vi "Edit user.vi"() -> ()   [LabVIEW 2017]
uses:
  <vilib>/Utility/error.llb/DialogType.ctl
  Globle/Cikautxo Intermix Login Details.vi
  Globle/Global 1.vi
panel:
  in  "Remove":bool
  out "error out":errorcluster
  out "Screen Index":i32
  in  "error in (no error)":errorcluster
  in  "User":bool
  in  "Authority":bool
  in  "Home":bool
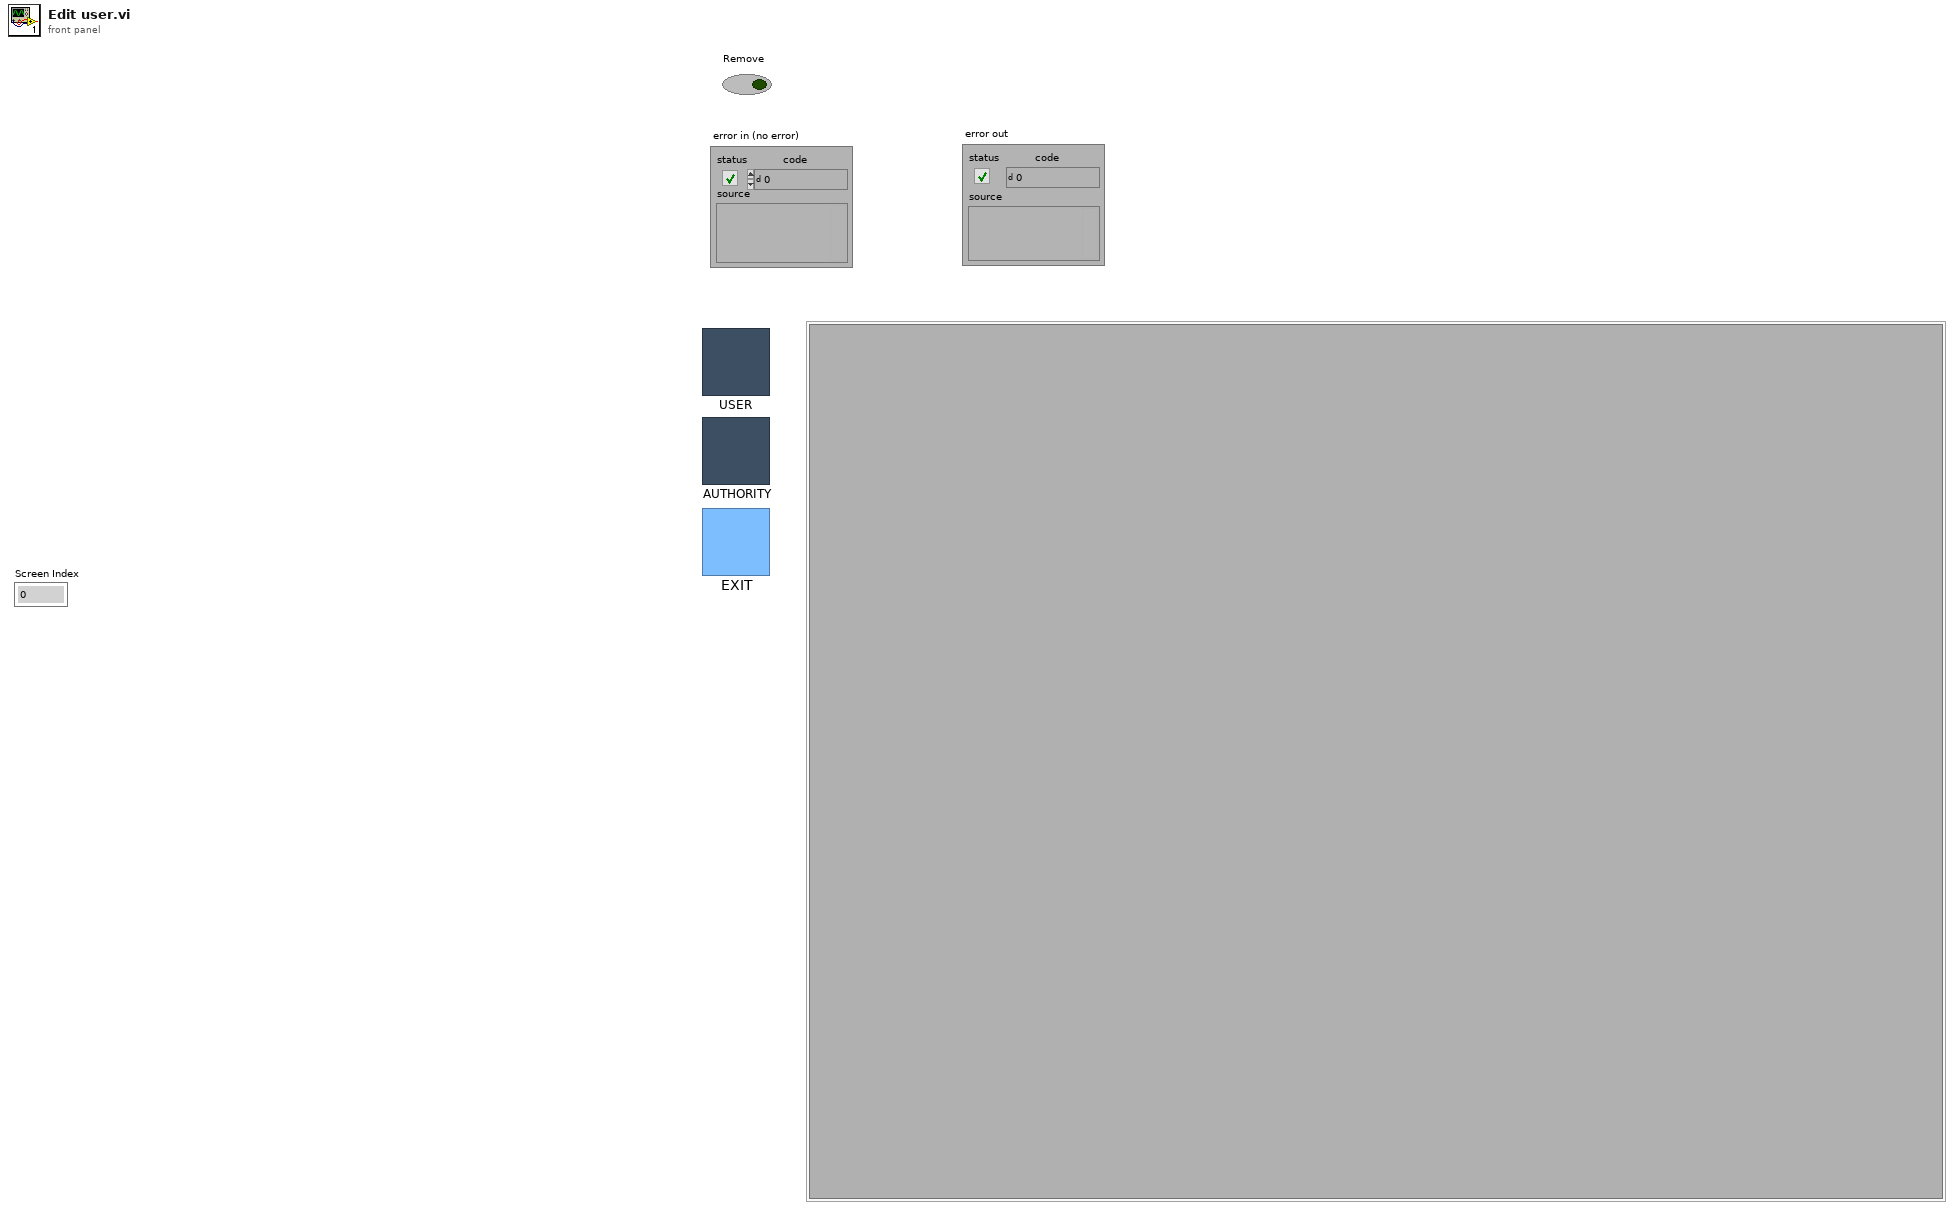
[diagram p1: front panel]
types:
  T1 = typedef "DialogType.ctl" = u16
  T2 = enum32{"invalid app kind", "Development System", "Run Time System", "Student Edition", "Embedded LabVIEW", "Evaluation", "Custom"}
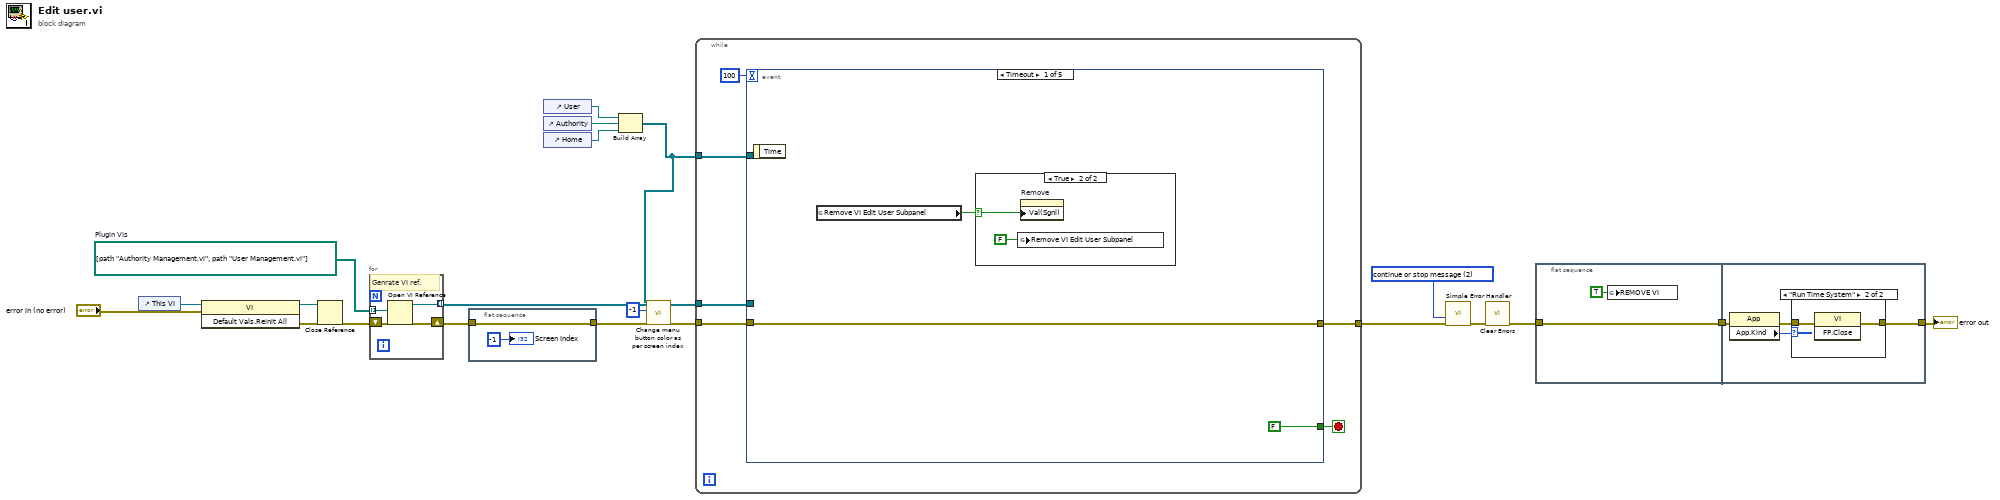
[diagram p0: block diagram]
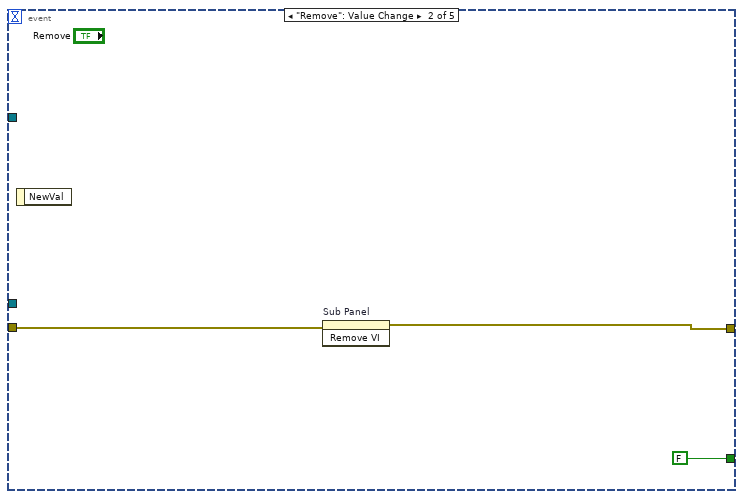
[diagram p4: hidden frame]
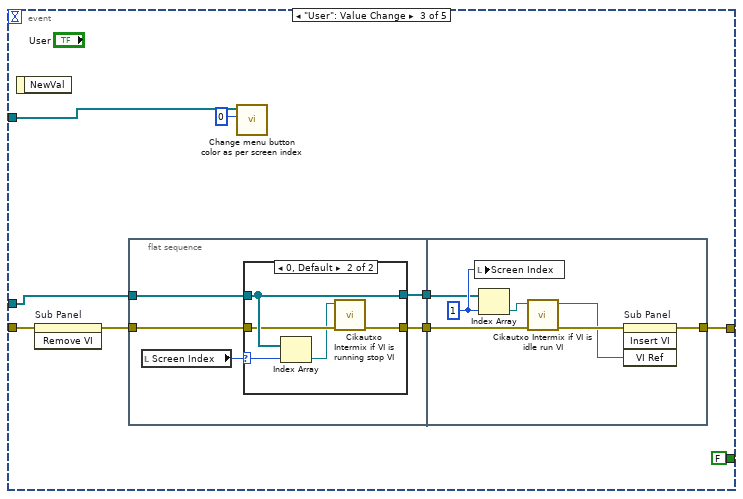
[diagram p5: hidden frame]
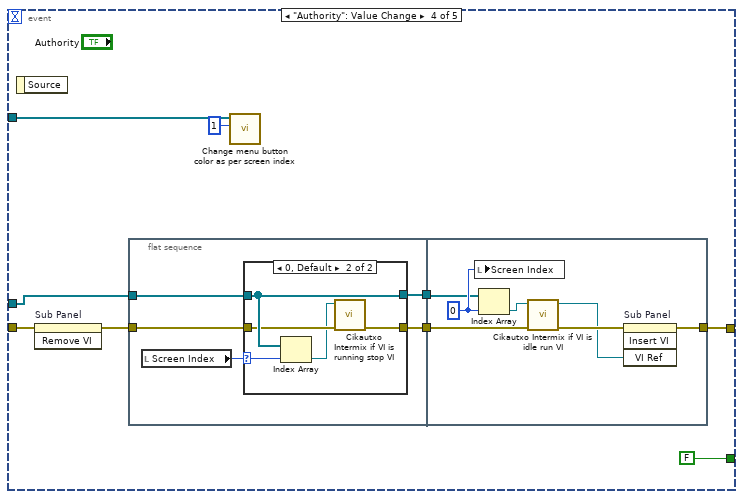
[diagram p7: hidden frame]
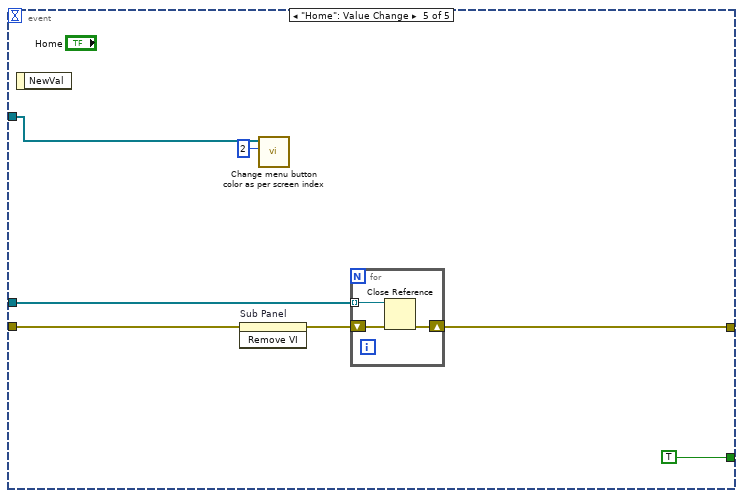
[diagram p9: hidden frame]
diagram:
  w10 = T1 2 items=["no dialog", "OK message", "continue or stop message", "OK message + warnings", "continue/stop + warnings"] ("type of dialog (OK msg:1)")
  w18 = path[] [path "Authority Management.vi", path "User Management.vi"]  # Plugin VIs
  n1 = control-ref of="This VI"() -> (w21:refnum<vi>)
  n2 = invoke class="VI" method="Default Vals.Reinit All"(reference=w21, error in="error in (no error)") -> (reference out=w19:refnum<vi>, error out=w20:errorcluster)  [unwired: 1 in, 1 out]
  n3 = Close Reference(reference=w19, error in (no error)=w20) -> (error out=w17:errorcluster)
  n4 = for {
    tunnel: w18 -> [w23] mode=indexing
    tunnel: [w24] -> w14 mode=indexing
    shift-right: [w25] -> w15
    shift-left: w17 -> [w22]
    # "Genrate VI ref."
    n5 = Open VI Reference(vi path=w23, error in (no error)=w22) -> (vi reference=w24:refnum<vi>, error out=w25:errorcluster)  [unwired: 4 in]
  }
  n6 = flat-sequence {
    tunnel: w15 -> [w27]
    tunnel: [w27] -> w2
    frame #0 {
      "Screen Index" <- -1 ("Screen Index")
    }
  }
  n7 = control-ref of="User"() -> (w6:refnum<vi>)
  n8 = control-ref of="Authority"() -> (w7:refnum<vi>)
  n9 = control-ref of="Home"() -> (w5:refnum<vi>)
  n10 = Build Array(w6, w7, w5) -> (w3:refnum<vi>[])
  n11 = call "Change menu button color as per screen index.vi"("error in (no error)"=w2, "Screen Index"=-1, "Array"=w3) -> ("error out"=w1:errorcluster)  [unwired: 8 in]
  n12 = while {
    tunnel: w1 -> [w31]
    tunnel: w14 -> [w29]
    tunnel: [w30] -> w9
    tunnel: w3 -> [w28]
    stop <- w32 stop-if-true
    n13 = event shown="[0] Timeout" {
      selector: _ -> [_ _ _ _ _]
      dyn-events: _ -> [_ _ _ _ _]
      timeout: 100 -> [_ _ _ _ _]
      tunnel: [FALSE FALSE FALSE FALSE TRUE] -> w32
      tunnel: [w35 w40 w45 w73 w100] -> w30
      tunnel: w31 -> [w35 w41 w47 w75 w101]
      tunnel: w29 -> [_ _ w46 w74 w102]
      tunnel: w28 -> [_ _ w43 w71 w99]
      event Timeout {
        n14 = event-data() -> ()  [unwired: 1 in, 1 out]
        n15 = global read "Cikautxo Intermix Login Details.vi" "Remove VI Edit User Subpanel"() -> (w34:bool)
        n16 = case shown="True" w34 {
          selector: w34 -> [_ w38]
          frame False {
          }
          frame True {
            n17 = global write "Cikautxo Intermix Login Details.vi" "Remove VI Edit User Subpanel"(FALSE ("Check")) -> ()
            n18 = property on="Remove" class="Bool (strict)"("Val(Sgnl)"=w38) -> ()  [unwired: 2 in, 2 out]
          }
        }
      }
      event "Remove": Value Change {
        n19 = event-data() -> ()  [unwired: 1 in, 1 out]
        n20 = invoke on="Sub Panel" class="SubPnl" method="Remove VI"(error in=w41) -> (error out=w40:errorcluster)  [unwired: 2 in, 2 out]
      }
      event "User": Value Change {
        n21 = event-data() -> ()  [unwired: 1 in, 1 out]
        n22 = invoke on="Sub Panel" class="SubPnl" method="Remove VI"(error in=w47) -> (error out=w48:errorcluster)  [unwired: 2 in, 2 out]
        n23 = flat-sequence {
          tunnel: w48 -> [w55]
          tunnel: w46 -> [w52]
          tunnel: [w54] -> w50
          tunnel: [w51] -> w49
          tunnel: [w67] -> w45
          tunnel: w50 -> [w66]
          tunnel: w49 -> [w68]
          frame #0 {
            n24 = local read "Screen Index"() -> (w53:i32)
            n25 = case shown="0, Default" w53 {
              selector: w53 -> [_ w62]
              tunnel: w55 -> [w57 w60]
              tunnel: [w57 w59] -> w54
              tunnel: w52 -> [w56 w61]
              tunnel: [w56 w61] -> w51
              frame -1 {
              }
              frame 0, Default {
                n26 = Index Array(array=w61, index=w62) -> (element=w58:refnum<vi>)
                n27 = call "Cikautxo Intermix if VI is running stop VI.vi"("error in (no error)"=w60, "VI in"=w58) -> ("error out"=w59:errorcluster)  [unwired: 8 in, 1 out]
              }
            }
          }
          frame #1 {
            w69 = 1 ("index")
            n28 = local write "Screen Index"(w69) -> ()
            n29 = Index Array(array=w68, index=w69) -> (element=w63:refnum<vi>)
            n30 = call "Cikautxo Intermix if VI is idle run VI.vi"("error in (no error)"=w66, "VI in"=w63) -> ("error out"=w65:errorcluster, "VI out"=w64:refnum<vi>)  [unwired: 8 in]
            n31 = invoke on="Sub Panel" class="SubPnl" method="Insert VI"(error in=w65, "VI Ref"=w64) -> (error out=w67:errorcluster)  [unwired: 2 in, 3 out]
          }
        }
        n32 = call "Change menu button color as per screen index.vi"("Screen Index"=0, "Array"=w43) -> ()  [unwired: 9 in, 1 out]
      }
      event "Authority": Value Change {
        n33 = event-data() -> ()  [unwired: 1 in, 1 out]
        n34 = invoke on="Sub Panel" class="SubPnl" method="Remove VI"(error in=w75) -> (error out=w76:errorcluster)  [unwired: 2 in, 2 out]
        n35 = flat-sequence {
          tunnel: w76 -> [w83]
          tunnel: w74 -> [w80]
          tunnel: [w82] -> w78
          tunnel: [w79] -> w77
          tunnel: [w95] -> w73
          tunnel: w78 -> [w94]
          tunnel: w77 -> [w96]
          frame #0 {
            n36 = local read "Screen Index"() -> (w81:i32)
            n37 = case shown="0, Default" w81 {
              selector: w81 -> [_ w90]
              tunnel: w83 -> [w85 w88]
              tunnel: [w85 w87] -> w82
              tunnel: w80 -> [w84 w89]
              tunnel: [w84 w89] -> w79
              frame -1 {
              }
              frame 0, Default {
                n38 = Index Array(array=w89, index=w90) -> (element=w86:refnum<vi>)
                n39 = call "Cikautxo Intermix if VI is running stop VI.vi"("error in (no error)"=w88, "VI in"=w86) -> ("error out"=w87:errorcluster)  [unwired: 8 in, 1 out]
              }
            }
          }
          frame #1 {
            w97 = 0 ("index")
            n40 = local write "Screen Index"(w97) -> ()
            n41 = Index Array(array=w96, index=w97) -> (element=w91:refnum<vi>)
            n42 = call "Cikautxo Intermix if VI is idle run VI.vi"("error in (no error)"=w94, "VI in"=w91) -> ("error out"=w93:errorcluster, "VI out"=w92:refnum<vi>)  [unwired: 8 in]
            n43 = invoke on="Sub Panel" class="SubPnl" method="Insert VI"(error in=w93, "VI Ref"=w92) -> (error out=w95:errorcluster)  [unwired: 2 in, 3 out]
          }
        }
        n44 = call "Change menu button color as per screen index.vi"("Screen Index"=1, "Array"=w71) -> ()  [unwired: 9 in, 1 out]
      }
      event "Home": Value Change {
        n45 = event-data() -> ()  [unwired: 1 in, 1 out]
        n46 = invoke on="Sub Panel" class="SubPnl" method="Remove VI"(error in=w101) -> (error out=w103:errorcluster)  [unwired: 2 in, 2 out]
        n47 = call "Change menu button color as per screen index.vi"("Screen Index"=2, "Array"=w99) -> ()  [unwired: 9 in, 1 out]
        n48 = for {
          shift-right: [w106] -> w100
          shift-left: w103 -> [w107]
          tunnel: w102 -> [w105] mode=indexing
          n49 = Close Reference(reference=w105, error in (no error)=w107) -> (error out=w106:errorcluster)
        }
      }
    }
  }
  n50 = call <vilib>:"Simple Error Handler.vi"("type of dialog (OK msg:1)"=w10, "error in (no error)"=w9) -> ("error out"=w13:errorcluster)  [unwired: 3 in, 4 out]
  n51 = call <vilib>:"Clear Errors.vi"("error in (no error)"=w13) -> ("error out"=w12:errorcluster)  [unwired: 5 in, 1 out]
  n52 = flat-sequence {
    tunnel: w12 -> [w109]
    tunnel: [w109] -> w8
    tunnel: [w110] -> w11
    tunnel: w8 -> [w111]
    frame #0 {
      n53 = global write "Global 1.vi" "REMOVE VI"(TRUE ("remove_VI")) -> ()
    }
    frame #1 {
      n54 = property class="App"(error in=w111) -> (error out=w112:errorcluster, "App.Kind"=w113:T2)  [unwired: 1 in, 1 out]
      n55 = case shown="\"Run Time System\"" w113 {
        tunnel: w112 -> [w114 w116]
        tunnel: [w114 w115] -> w110
        frame Default {
        }
        frame "Run Time System" {
          n56 = invoke class="VI" method="FP.Close"(error in=w116) -> (error out=w115:errorcluster)  [unwired: 2 in, 2 out]
        }
      }
    }
  }
  "error out" <- w11
